vi "add attributes.vi"(8 "error in (no error)":errorcluster, 9 "Variant":variant, 10 "Item Indent":i32, 11 "Items in":T1(array[cluster])) -> (0 "error out":errorcluster, 3 "Items out":T1(array[cluster]))   [LabVIEW 2016]
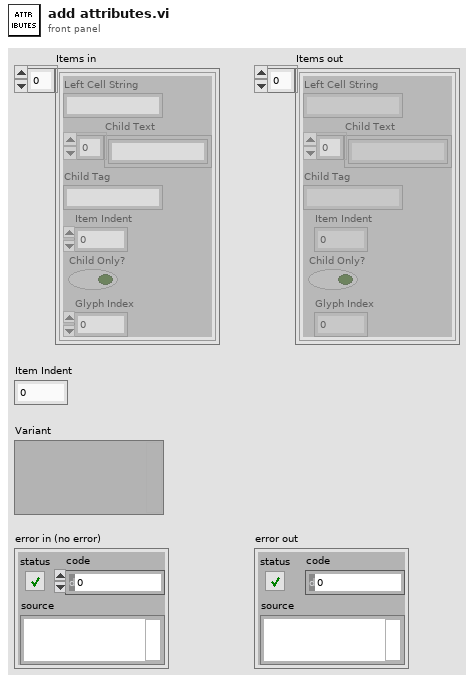
[diagram p1: front panel]
types:
  T1 = cluster{"Left Cell String":string, "Child Text":string[], "Child Tag":string, "Item Indent":i32, "Child Only?":bool, "Glyph Index":i32}[]
  T2 = cluster{"Left Cell String":string, "Child Text":string[], "Child Tag":string, "Item Indent":i32, "Child Only?":bool, "Glyph Index":i32}
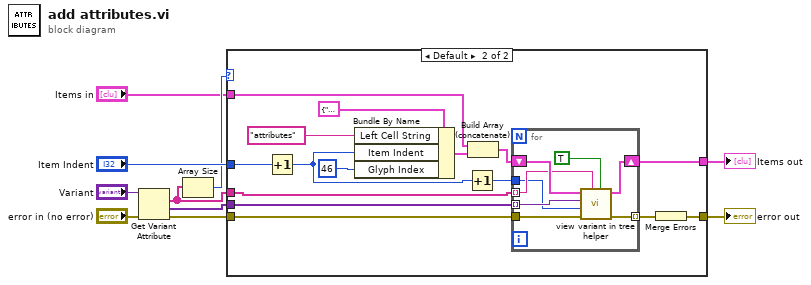
[diagram p0: block diagram]
diagram:
  n1 = Get Variant Attribute(Variant="Variant", error in="error in (no error)") -> (names=w5:string[], values=w2:variant[], error out=w8:errorcluster)  [unwired: 2 in, 1 out]
  n2 = Array Size(array=w5) -> (size(s)=w6:i32)
  n3 = case shown="Default" w6 {
    tunnel: w2 -> [_ w27]
    tunnel: "Items in" -> [w12 w24]
    tunnel: [w12 w26] -> w4
    tunnel: w5 -> [_ w25]
    tunnel: "Item Indent" -> [_ w23]
    tunnel: w8 -> [w11 w15]
    tunnel: [w11 w13] -> w9
    frame 0 {
    }
    frame Default {
      n4 = Increment(x=w23) -> (x+1=w19:i32)
      n5 = Bundle By Name(cluster=T2 {"Left Cell String"="", "Child Text"=[], "Child Tag"="", "Item Indent"=0, "Child Only?"=FALSE, "Glyph Index"=0} ("Item"), "Left Cell String"="attributes", "Item Indent"=w19, "Glyph Index"=46) -> (w18:T2)
      n6 = Increment(x=w19) -> (x+1=w22:i32)
      n7 = Build Array (concatenate)(w24, w18) -> (w17:T1)
      n8 = for {
        tunnel: w27 -> [w35] mode=indexing
        shift-right: [w33] -> w26
        shift-left: w17 -> [w34]
        tunnel: w25 -> [w32] mode=indexing
        tunnel: w22 -> [w30]
        tunnel: w15 -> [w29]
        tunnel: [w28] -> w14 mode=indexing
        n9 = call "view variant in tree helper.vi"("is attribute?"=TRUE, "name"=w32, "error in (no error)"=w29, "Item Indent"=w30, "Variant"=w35, "Items"=w34) -> ("error out"=w28:errorcluster, "Items out"=w33:T1)  [unwired: 4 in]
      }
      n10 = Merge Errors(w14) -> (w13:errorcluster)
    }
  }
  "error out" <- w9
  "Items out" <- w4
